vi "Test signal driver.vi"() -> ()   [LabVIEW 2011]
uses:
  <vilib>/Analysis/NI_AALBase.lvlib
  <vilib>/Analysis/NI_AALPro.lvlib
panel:
  out "FFT":dbl[](graph)
  out "DWT":dbl[][](graph)
  out "Input":dbl[](graph)=[-0.5000127629647003, 1.2796838611483974, 0.5937124283560136, 0.5309320916346331, 1.4223053563604449, 1.2489084435941482, 1.7315855041682093, 1.6935128596863291, 1.6633580540558746, 1.3862552469354905, 1.270049445967233, 1.2736334757288643, 0.6513322825140464, 0.4699755587592019, -0.273741362451403, 0.22184289765792553, -0.2473854377462329, 0.048893172288155484, 0.4618719819328262, 0.5429975905265254, 0.9017938655192154, -0.07192492403286277, 0.3779135726974272, 1.4502865547816253, 1.0978203700063507, 0.9801965661514067, 1.2916933391002858, 1.1035852590549189, 2.206610443534035, 3.016412847165209, 1.2413301982493525, 1.232689439607797, 0.6523583382701508, 1.0254242924180323, 0.5813130567537816, -0.24124908287976732, -0.7159192016368268, 0.24137095643561426, -0.1279235037796585, -0.9412278577655288, -0.7087603766718478, -1.8430901915956481, -1.6388082455320028, -1.201566813194174, -0.8784399388055497, -0.28376975711089086, -0.6075199939823219, -0.5501335332090698, -0.5530286923668382, 1.1697843139953814, -0.5760301968924436, 0.26155519993404375, 0.4260213077676267, 0.3759513491427683, 0.9514901795779617, -0.5974146641203695, -1.4811211881928026, -1.0021694843491094, -1.3200075867211463, -1.1068607473965204, -1.2996495457465564, -1.7753060271602863, -1.4414123413299038, -1.6094969046652263, -1.1403022326882128, -1.802495214781427, -1.4123093715448949, -1.5498709526420371, -2.0711602533086237, -0.1966184374897615, -0.6915269419688514, -0.3785227402616656, 0.285848507344953, 0.5730369971933875, 0.7081694081145811, 0.6997816198757186, 0.8886056242787759, 1.2446220340587935, 0.8700317941664627, 0.5880183822007822, 1.157714836669122, 0.6618564328548545, 0.5141719863913986, -0.5459915196430574, 0.0801303369281342, 0.680646253198879, 0.16144046397273093, -0.5424918950443567, -0.6425117419109855, -0.3668391547843539, 0.2622369779717524, 0.5864907689036731, 0.9526676902201219, 1.683627123619996, 0.7114879292439336, 1.5417210013422307, 1.6495816772499554, 1.8463914157582784, 2.1892544479248066, 0.40561643516991575, 2.405601581452003, 1.5782644696369657, 0.8322776859714187, 1.4629902060359106, 0.34704369373357924, 0.6819193147600059, 0.43936367021176237, 0.49484155367105, -0.8859376462289339, -1.4101168430623696, -0.19765566927615108, -0.2648210267887836, -0.6830505255875035, -0.1191748520697185, -0.791590843997305, 0.351664500973753, -0.17584921854790866, 0.508423318394116, 1.3873289592136937, 0.8726979966135919, 0.8887404118383735, 0.16708557897423149, 1.632833188197985, 1.3166999784134585, 0.07537202024923084, -1.2276159841624492, -0.2593394149163327, -0.9268573898646847, -1.1726648916606042, -0.7643771645334025, -1.9805922907415638, -1.9468264391956134, -1.6887415986752732, -1.5040032804279861, -1.749426521849975, -1.801945440779746, -1.0756602373676727, -1.0863261144243748, -0.9551720157826609, 0.045749620223788146, -0.3530223383886968, -0.13728053480549596, -0.23530161771219515, -0.061269154291558436, -0.005315358416301819, 1.0550329037195083, -0.16425774229681445, 0.17300410146004574, -0.28013985192705804, 0.6974397016324949, 0.36697578116641605, -0.9975038478504098, -0.512598386991706, -0.452668695602905, -1.0052350088390514, -0.94817135497532, -0.5962292570599292, -0.5003813018662504, -0.7358223413619732, -1.485830285820211, -0.09678940099145245, -0.05442724629326812, 0.86816296006954, 0.5896001204127242, 1.283025264829412, 1.701074242659662, 1.0148819892978307, 2.0812646183099055, 1.6933780829673657, 2.04511978300373, 1.8395766911824878, 1.684072004120416, 0.8430262017882867, 0.6313790675747752, 0.3345159329153772, 0.8175483319611759, -0.3846432673544279, -0.046264617628114735, -0.6146982490250662, -0.1470227806811807, 0.49470528661098134, 1.0438903706793439, 0.8673097243747179, 0.18783928636522484, 0.3474223065494467, 0.37708025769773235, 0.8366493324556737, 0.4853962830904289, 1.6192425267067079, 0.7356835142223674, 0.9095081412263764, 1.1721879059743867, 2.1003634808603193, 0.6675291239573387, 0.11081024357856328, 0.5234456706258938, 0.17646995736890683, -0.5693012925041976, -0.9520557532037401, -0.6751511586815269, -1.3453121434416628, -1.4193143758393447, -1.7108023631718519, -0.5639714541177085, -1.4495648776431336, -2.411993525529935, -1.9546484024306294, -0.8070082826929408, -0.8229886053118711, -0.6966261895184009, -0.7474105417727501, -0.84268224198029, 0.7739312769773671, -0.13939040582089135, 0.417012260105766, 0.029010557074562238, -0.286309797547011, -0.6816789931827869, -0.19902252819299204, -0.5184339890571382, -0.23383189750414968, -2.0160332999537087, -1.3799737672680892, -1.9950305490993443, -1.2149129687148752, -2.0270815534776396, -0.7481511099540619, -1.4027085154660301, -0.9354033417647762, -0.9933583225462439, -0.036274334062592783, -0.3361082316605092, 0.6825454948091977, 0.3660816137026882, 0.8813578689775212, 1.0817901741676437, 1.2597726428651583, 0.7515184455082198, 2.3968186806520153, 1.5320671124289276, 0.4834528954058991, 2.486089852531925, 0.8355426344785433, 1.438026123504268, 0.9359731389249584, 0.5333466928716777, 0.051309748362072916, 0.7811687532662156, 0.9775285737445218, -0.42721767541556044, -0.16093932075774586, -0.9981876134617821, 0.23768020039423732, 0.8014295235123942, 0.24856173188053987, 0.7318854397725008]
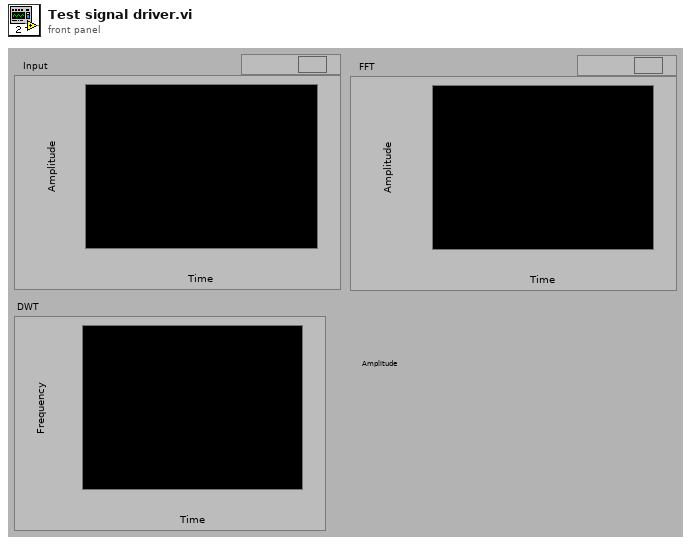
[diagram p1: front panel]
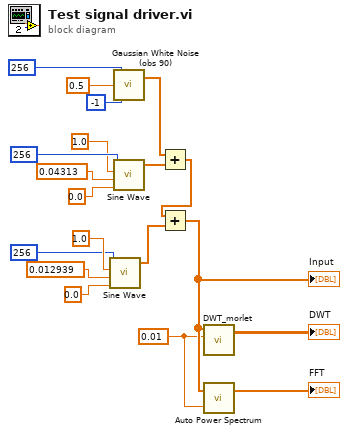
[diagram p0: block diagram]
diagram:
  w1 = 0.01 ("phase in")
  n1 = call <vilib>:"Sine Wave.vi"("samples"=256, "amplitude"=1.0, "frequency"=0.012939 ("f"), "phase in"=0.0) -> ("sine wave"=w12:dbl[])  [unwired: 1 in, 2 out]
  n2 = call <vilib>:"Gaussian White Noise (obs 90).vi"("seed"=-1, "standard deviation"=0.5, "samples"=256) -> ("Gaussian noise pattern"=w4:dbl[])  [unwired: 1 out]
  n3 = call <vilib>:"Sine Wave.vi"("samples"=256, "amplitude"=1.0, "frequency"=0.04313 ("f"), "phase in"=0.0) -> ("sine wave"=w5:dbl[])  [unwired: 1 in, 2 out]
  n4 = Add(x=w4, y=w5) -> (x+y=w7:dbl[])
  n5 = Add(x=w7, y=w12) -> (x+y=w3:dbl[])
  "Input" <- w3
  n6 = call "DWT_morlet.vi"("dt"=w1, "1D Real input"=w3) -> ("Wavelet plot"=→"DWT":dbl[][])  [unwired: 5 in]
  n7 = call <vilib>:"Auto Power Spectrum.vi"("dt"=w1, "Signal (V)"=w3) -> ("Power Spectrum (V^2 rms)"=→"FFT":dbl[])  [unwired: 1 out]
